vi "create.vi"(8 "error in (no error)":errorcluster, 9 "manager_daemon":refnum<class "manager_daemon.lvclass">, 10 "issue directory":path, 11 "volume directory":path) -> (0 "error out":errorcluster, 3 "ComicVine_manager out":refnum<class "ComicVine_manager.lvclass">)   [LabVIEW 2024, in "ComicVine_manager.lvclass"]
uses:
  ComicVine_manager.lvclass
  states--enum.ctl
  status--cluster.ctl
  private/queue.message--cluster.ctl
  ComicVine_manager.lvclass/ComicVine_manager.ctl
  <userlib>/_OpenG.lib/file/file.llb/openg_file.lvlib
  comic_manager/manager_daemon/manager_daemon.lvclass
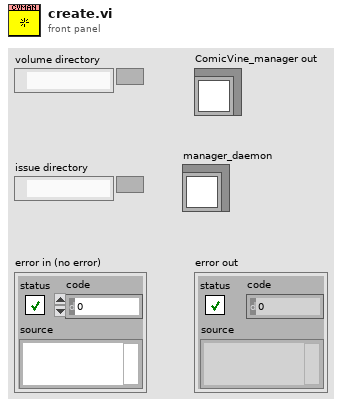
[diagram p1: front panel]
types:
  T1 = typedef "ComicVine_manager.lvclass/queue.message--cluster.ctl" = cluster{"cmd":T2, "data":variant}
  T2 = typedef "ComicVine_manager.lvclass/states--enum.ctl" = enum16{"start", "running", "start timer", "update file", "set directories", "wait", "shutdown"}
  T3 = typedef "ComicVine_manager.lvclass/status--cluster.ctl" = cluster{"files in queue":i32, "in jail?":bool, "current state":string, "time left (s)":dbl, "iteration":i32, "error status":errorcluster, "log file":path}
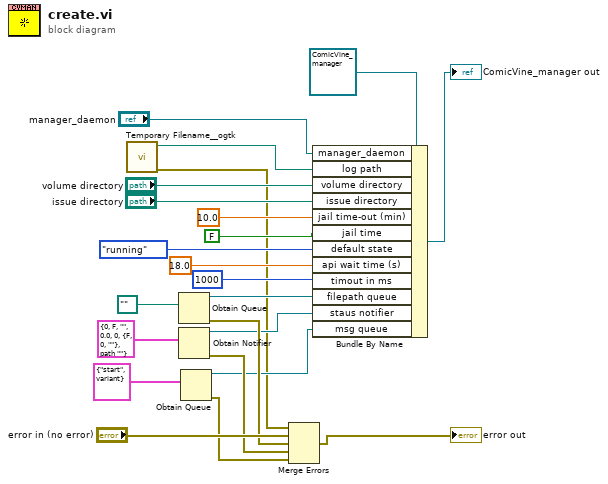
[diagram p0: block diagram]
diagram:
  n1 = call <userlib>:"Temporary Filename__ogtk.vi"() -> ("error out"=w2:errorcluster, "file in tmp dir"=w3:path)  [unwired: 6 in]
  n2 = Obtain Queue(element data type=path "") -> (queue out=w21:refnum<queue>, error out=w15:errorcluster)  [unwired: 4 in, 1 out]
  n3 = Obtain Notifier(notification data type=T3 {"files in queue"=0, "in jail?"=FALSE, "current state"="", "time left (s)"=0.0, "iteration"=0, "error status"={"status"=FALSE, "code"=0, "source"=""}, "log file"=path ""} ("status")) -> (notifier out=w12:refnum<notifier>, error out=w11:errorcluster)  [unwired: 3 in, 1 out]
  n4 = Obtain Queue(element data type=T1 {"cmd"=enum."start", "data"=variant} ("message")) -> (queue out=w5:refnum<queue>, error out=w4:errorcluster)  [unwired: 4 in, 1 out]
  n5 = Merge Errors(w2, "error in (no error)", w15, w11, w4) -> (→"error out":errorcluster)
  n6 = Bundle By Name(cluster=refnum<class "ComicVine_manager.lvclass"> refnum ("ComicVine_manager.lvclass"), "manager_daemon"="manager_daemon", "log path"=w3, "volume directory"="volume directory", "issue directory"="issue directory", "jail time-out (min)"=10.0, "jail time"=FALSE, "default state"=states--enum."running", "api wait time (s)"=18.0 ("jail time-out (min)"), "timout in ms"=1000, "filepath queue"=w21, "staus notifier"=w12, "msg queue"=w5) -> (→"ComicVine_manager out":refnum<class "ComicVine_manager.lvclass">)
